vi "Run_4_of_6_Tests.vi"() -> ()   [LabVIEW 2019]
uses:
  <vilib>/Rock Robotics/WPI/ThirdParty/JAS_Junk/TrajLib/Trajectory_Library.lvlib
panel:
  out "String":string
  out "Vision Utilities":bool
  out "Trajectory Generate":bool
  out "Trajectory Transform":bool
  out "Units":bool
  out "All Tests Finished":bool
  out "Trajectory JSON":bool
  out "Trapezoid Profile":bool
  out "Unscented Kalman Filter":bool
  out "Twist2d":bool
  out "Translation2d":bool
  out "Transform2d":bool
  # "FORMAL TRAJECTORY / CONTROL LIBRARY TEST PROCEDURE"
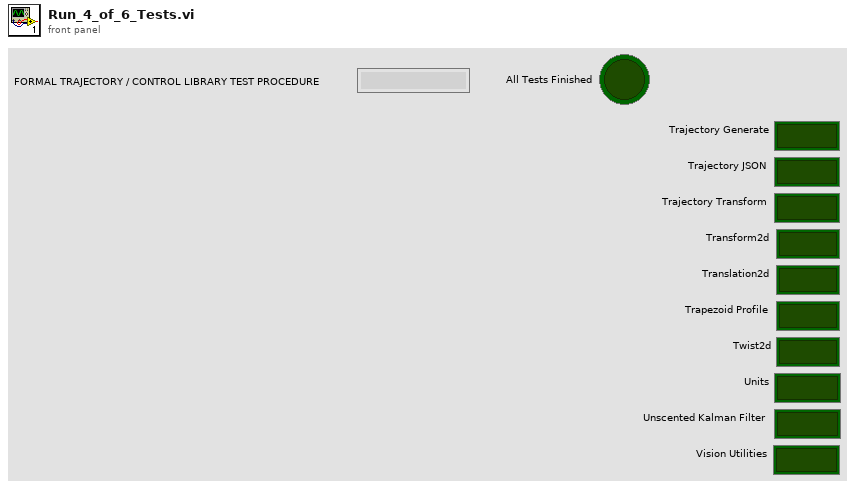
[diagram p1: front panel]
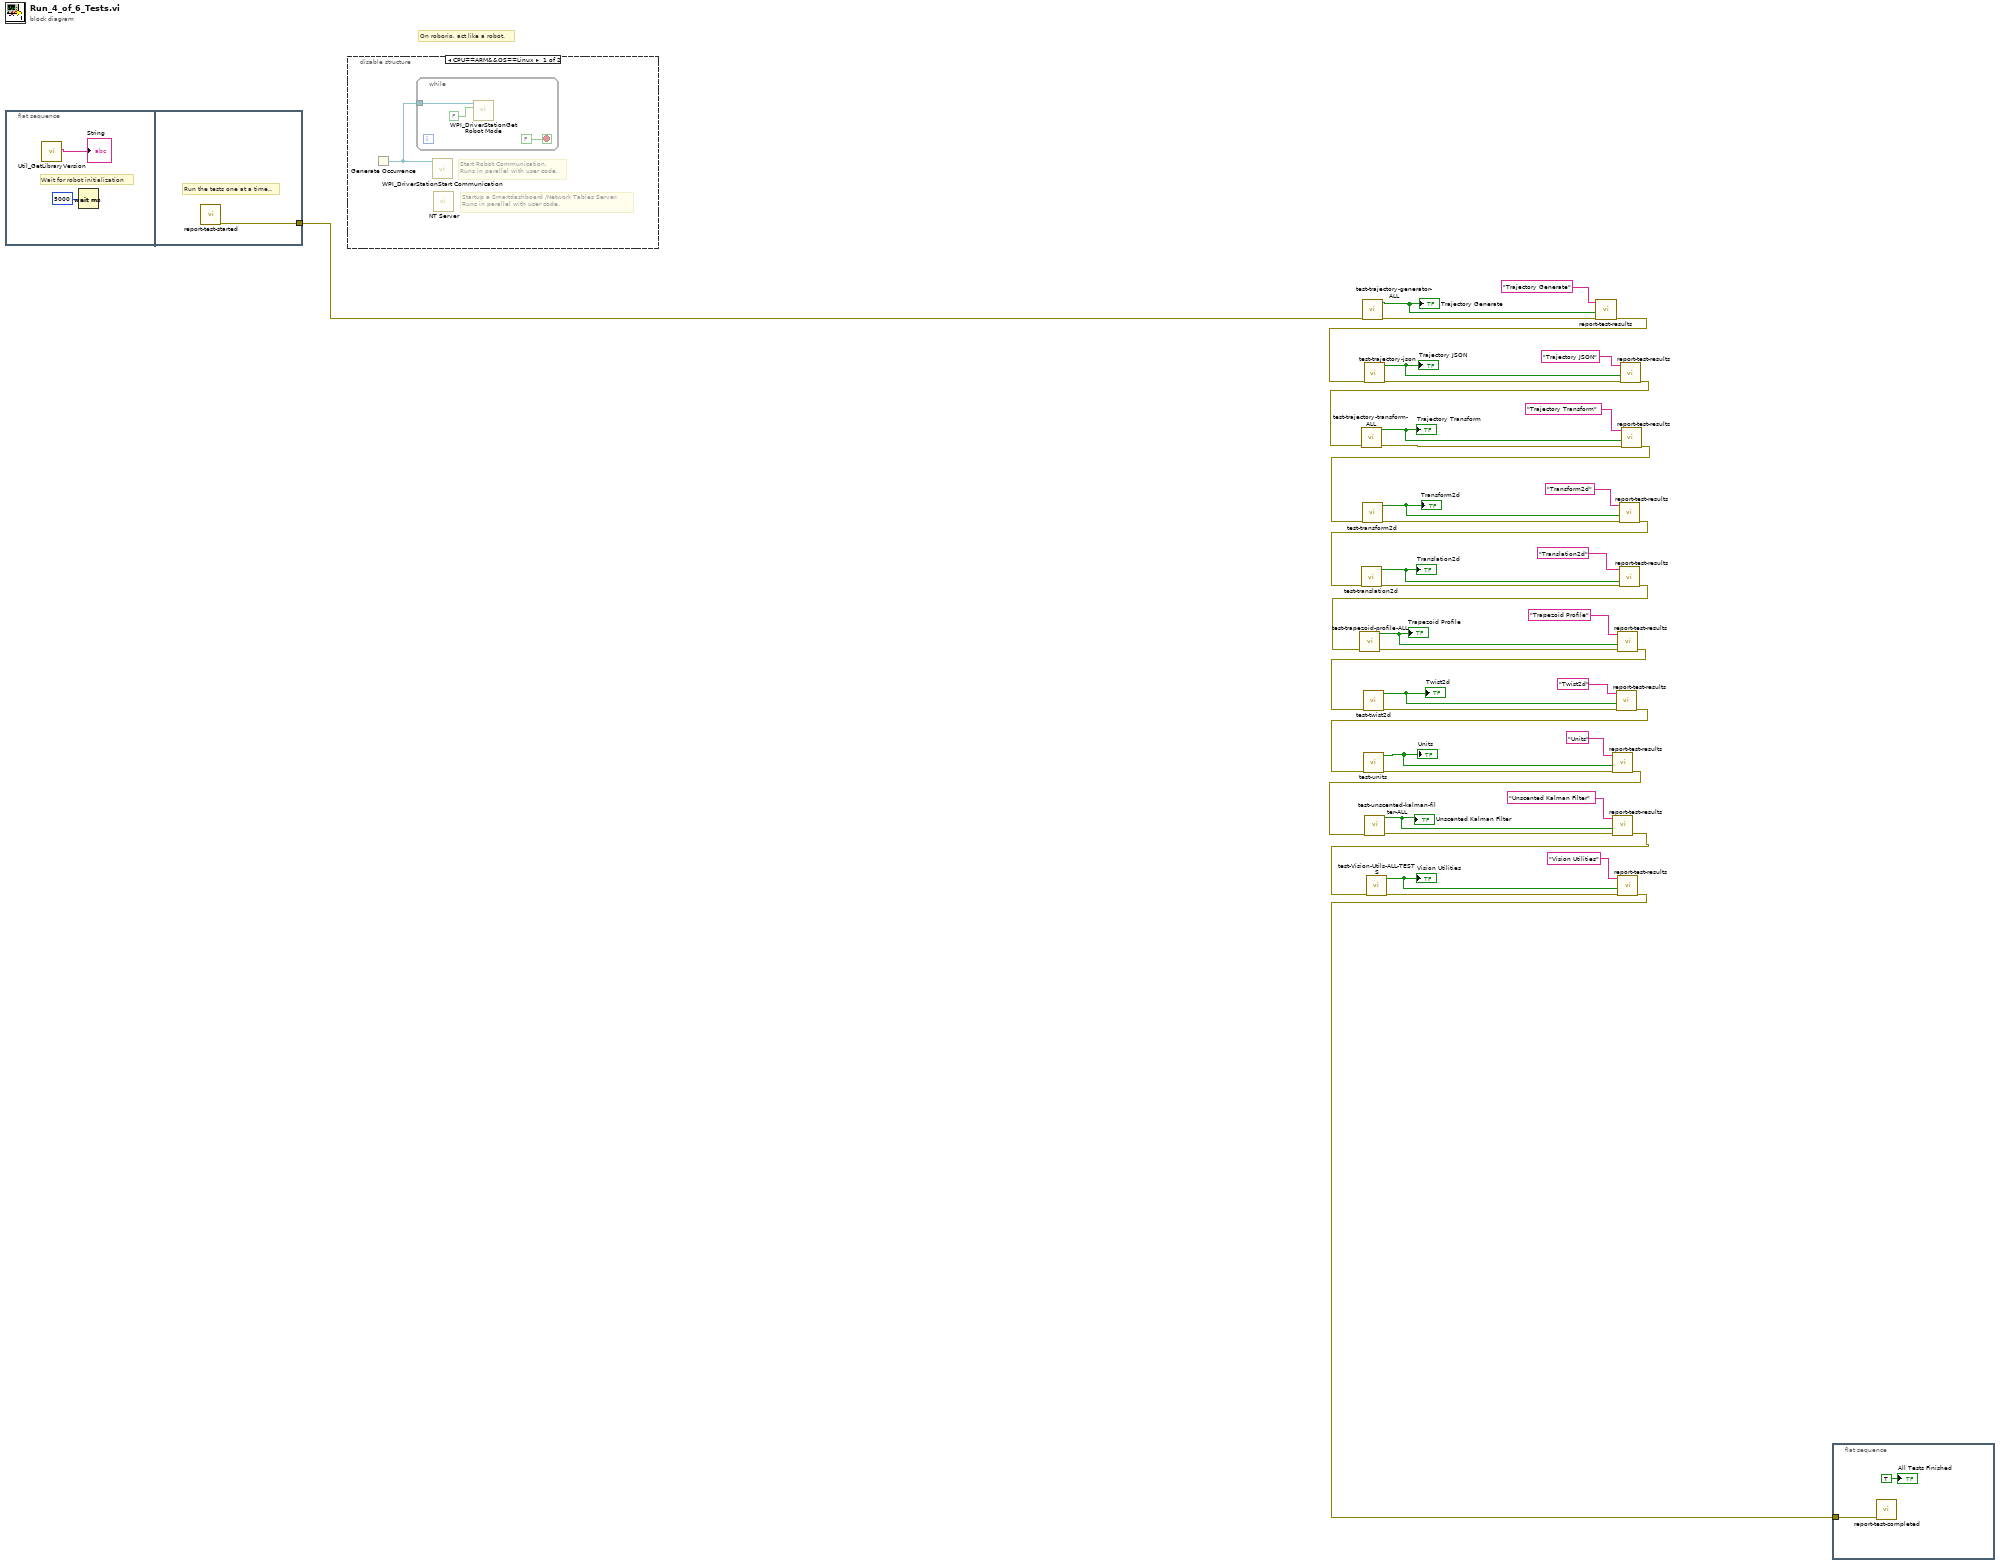
[diagram p0: block diagram]
diagram:
  # "On roborio, act like a robot."
  n1 = flat-sequence {
    tunnel: [w44] -> w6
    frame #0 {
      # "Wait for robot initialization"
      n2 = call <vilib>:"Util_GetLibraryVersion.vi"() -> ("TrajLibVersion"=→"String":string)  [unwired: 11 in]
      n3 = Wait (ms)(milliseconds to wait=u32 5000) -> ()  [unwired: 1 out]
    }
    frame #1 {
      # "Run the tests one at a time.."
      n4 = call "report-test-started.vi"() -> ("error out"=w44:errorcluster)  [unwired: 11 in]
    }
  }
  n5 = disable-structure shown="CPU==ARM&&OS==Linux" {
    frame condition #0 {
      # "Startup a Smartdashboard /Network Tables Server.\nRuns in parallel with user code."
      # "Start Robot Communication.\nRuns in parallel with user code."
      n6 = Generate Occurrence() -> (w45:refnum<k4>)
      n7 = while {
        tunnel: w45 -> [w48]
        stop <- FALSE stop-if-true
        n8 = call <vilib>:"WPI_DriverStationGet Robot Mode.vi"("Finish"=FALSE, "DS Occurrence"=w48) -> ()  [unwired: 10 out]
      }
      n9 = call <vilib>:"WPI_DriverStationStart Communication.vi"("occurrence"=w45) -> ()  [unwired: 2 in, 9 out]
      n10 = call <vilib>:"NT Server.vi"() -> ()  [unwired: 12 in]
    }
    frame condition #1 (active) {
    }
  }
  n11 = call "test-trajectory-generator-ALL.vi"("error in (no error)"=w6) -> ("error out"=w23:errorcluster, "ALL TESTS PASSED"=w40:bool)  [unwired: 9 in]
  "Trajectory Generate" <- w40
  n12 = call "report-test-results.vi"("error in (no error)"=w23, "TestPassed"=w40, "Test Name"="Trajectory Generate") -> ("error out"=w7:errorcluster)  [unwired: 8 in]
  n13 = call "test-trajectory-json.vi"("error in (no error)"=w7) -> ("error out 2"=w17:errorcluster, "ALL TESTS PASSED"=w32:bool)  [unwired: 9 in]
  "Trajectory JSON" <- w32
  n14 = call "report-test-results.vi"("error in (no error)"=w17, "TestPassed"=w32, "Test Name"="Trajectory JSON") -> ("error out"=w13:errorcluster)  [unwired: 8 in]
  n15 = call "test-trajectory-transform-ALL.vi"("error in (no error)"=w13) -> ("error out 2"=w16:errorcluster, "Test Passed"=w31:bool)  [unwired: 9 in]
  "Trajectory Transform" <- w31
  n16 = call "report-test-results.vi"("error in (no error)"=w16, "TestPassed"=w31, "Test Name"="Trajectory Transform") -> ("error out"=w12:errorcluster)  [unwired: 8 in]
  n17 = call "test-transform2d.vi"("error in (no error)"=w12) -> ("error out"=w18:errorcluster, "All PASSED"=w30:bool)  [unwired: 9 in]
  "Transform2d" <- w30
  n18 = call "report-test-results.vi"("error in (no error)"=w18, "TestPassed"=w30, "Test Name"="Transform2d") -> ("error out"=w11:errorcluster)  [unwired: 8 in]
  n19 = call "test-translation2d.vi"("error in (no error)"=w11) -> ("error out"=w19:errorcluster, "All PASSED"=w29:bool)  [unwired: 9 in]
  "Translation2d" <- w29
  n20 = call "report-test-results.vi"("error in (no error)"=w19, "TestPassed"=w29, "Test Name"="Translation2d") -> ("error out"=w10:errorcluster)  [unwired: 8 in]
  n21 = call "test-trapezoid-profile-ALL.vi"("error in (no error)"=w10) -> ("error out"=w20:errorcluster, "All TEsts passed"=w28:bool)  [unwired: 9 in]
  "Trapezoid Profile" <- w28
  n22 = call "report-test-results.vi"("error in (no error)"=w20, "TestPassed"=w28, "Test Name"="Trapezoid Profile") -> ("error out"=w9:errorcluster)  [unwired: 8 in]
  n23 = call "test-twist2d.vi"("error in (no error)"=w9) -> ("error out"=w21:errorcluster, "All PASSED"=w27:bool)  [unwired: 9 in]
  "Twist2d" <- w27
  n24 = call "report-test-results.vi"("error in (no error)"=w21, "TestPassed"=w27, "Test Name"="Twist2d") -> ("error out"=w8:errorcluster)  [unwired: 8 in]
  n25 = call "test-units.vi"("error in (no error)"=w8) -> ("error out"=w15:errorcluster, "All Tests Passed"=w26:bool)  [unwired: 9 in]
  "Units" <- w26
  n26 = call "report-test-results.vi"("error in (no error)"=w15, "TestPassed"=w26, "Test Name"="Units") -> ("error out"=w14:errorcluster)  [unwired: 8 in]
  n27 = call "test-unscented-kalman-filter-ALL.vi"("error in (no error)"=w14) -> ("error out"=w22:errorcluster, "All Tests Passed"=w24:bool)  [unwired: 9 in]
  "Unscented Kalman Filter" <- w24
  n28 = call "report-test-results.vi"("error in (no error)"=w22, "TestPassed"=w24, "Test Name"="Unscented Kalman Filter") -> ("error out"=w2:errorcluster)  [unwired: 8 in]
  n29 = call "test-Vision-Utils-ALL-TESTS.vi"("error in (no error)"=w2) -> ("error out"=w4:errorcluster, "All Passed"=w3:bool)  [unwired: 9 in]
  "Vision Utilities" <- w3
  n30 = call "report-test-results.vi"("error in (no error)"=w4, "TestPassed"=w3, "Test Name"="Vision Utilities") -> ("error out"=w1:errorcluster)  [unwired: 8 in]
  n31 = flat-sequence {
    tunnel: w1 -> [w49]
    frame #0 {
      n32 = call "report-test-completed.vi"("error in (no error)"=w49) -> ()  [unwired: 10 in, 1 out]
      "All Tests Finished" <- TRUE ("All Tests Finished")
    }
  }
